vi "Create DVR.vi"(5 "Actor Ref":refnum<vi>, 6 "timeout (10000)":i32=10000, 7 "client handle":refnum<k1>, 8 "error in (no error)":errorcluster, 9 "output file":path, 10 "file size":i64, 11 "GET Async in":refnum<class "GET Async.lvclass">) -> (0 "error out":errorcluster, 3 "HTTP GET Async ref":refnum<data-value>)   [LabVIEW 2019, in "HTTP Client Extensions.lvlib" / "GET Async.lvclass"]
uses:
  GET Async.lvclass
  GET Async.lvclass/GET Async.ctl
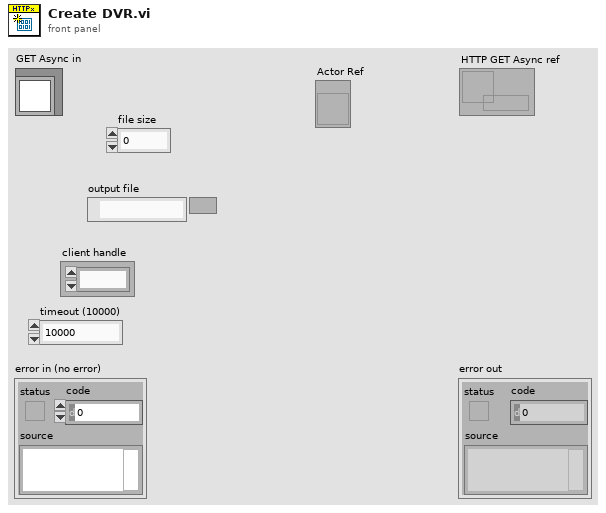
[diagram p1: front panel]
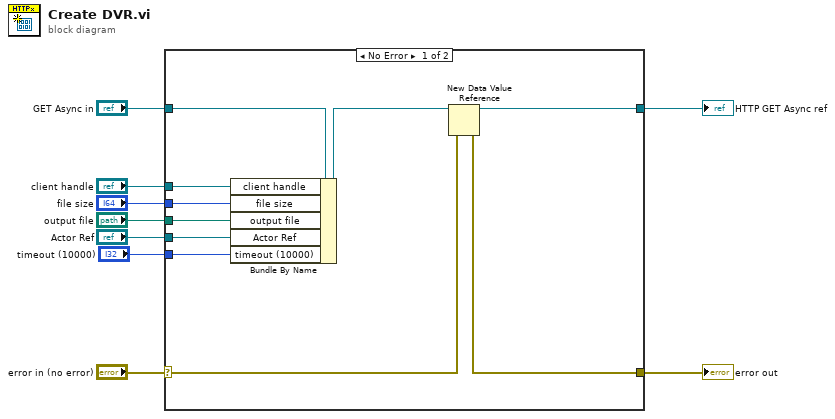
[diagram p0: block diagram]
diagram:
  n1 = case shown="No Error" "error in (no error)" {
    selector: "error in (no error)" -> [w18 w20]
    tunnel: [w17 w20] -> w8
    tunnel: [w19 _] -> w6
    tunnel: "GET Async in" -> [w16 _]
    tunnel: "client handle" -> [w14 _]
    tunnel: "file size" -> [w13 _]
    tunnel: "output file" -> [w12 _]
    tunnel: "Actor Ref" -> [w11 _]
    tunnel: "timeout (10000)" -> [w10 _]
    frame No Error {
      n2 = Bundle By Name(cluster=w16, "client handle"=w14, "file size"=w13, "output file"=w12, "Actor Ref"=w11, "timeout (10000)"=w10) -> (w15:refnum<class "GET Async.lvclass">)
      n3 = New Data Value Reference(data value=w15, error in=w18) -> (data value reference=w19:refnum<data-value>, error out=w17:errorcluster)
    }
    frame Error {
    }
  }
  "error out" <- w8
  "HTTP GET Async ref" <- w6
